vi "launcher.vi"() -> ()   [LabVIEW 2023]
uses:
  Libraries/SinglePhotonInterferenceUI/SinglePhotonInterferenceUI/SinglePhotonInterferenceUI.lvclass
  Libraries/SPIController/SPIController/SPIController.lvclass
  TranslationStage_UI/TranslationStage_UI/TranslationStageUI.lvclass
  <vilib>/ActorFramework/Actor/Actor.lvclass
panel:
  in  "Control":enum16{"Multiharp", "SPI", "Stepper Motor"}(ring)=enum."Stepper Motor"
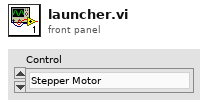
[diagram p1: front panel]
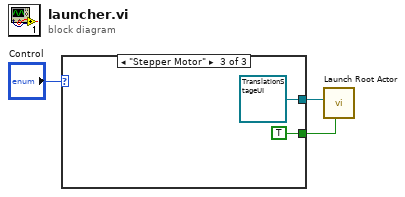
[diagram p0: block diagram]
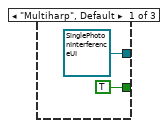
[diagram p2: hidden frame]
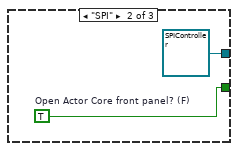
[diagram p3: hidden frame]
diagram:
  n1 = case shown="\"Stepper Motor\"" "Control" {
    tunnel: [TRUE ("Open Actor Core front panel? (F)") w7 TRUE ("Open Actor Core front panel? (F)")] -> w2
    tunnel: [refnum<class "SinglePhotonInterferenceUI.lvclass"> refnum ("SinglePhotonInterferenceUI.lvlib:SinglePhotonInterferenceUI.lvclass") refnum<class "SPIController.lvclass"> refnum ("SPIController.lvlib:SPIController.lvclass") refnum<class "TranslationStageUI.lvclass"> refnum ("TranslationStageUI.lvclass")] -> w1
    frame "Multiharp", Default {
    }
    frame "SPI" {
      w7 = TRUE  # Open Actor Core front panel? (F)
    }
    frame "Stepper Motor" {
    }
  }
  n2 = call <vilib>:"Launch Root Actor.vi"("Open Actor Core front panel? (F)"=w2, "Actor"=w1) -> ()  [unwired: 8 in, 2 out]
